vi "Analog Servo FPGA.vi"(9 "stop":bool) -> (1 "Clock":bool, 2 "Position Command":fxp<+/-,32,32>)   [LabVIEW 2012]
uses:
  <vilib>/Platform/TimedLoop/XDataNode/timing_clust.ctl
  <vilib>/Platform/TimedLoop/XDataNode/nitl_modes.ctl
  <vilib>/Platform/TimedLoop/XDataNode/wakeup.ctl
  <vilib>/rvi/Emulation/niFpgaSctlEmulationRegisterWithScheduler.vi
  <vilib>/rvi/eio/common/nirviEmuTemplateMethod_errors.vi
  <vilib>/rvi/Emulation/niFpgaSctlEmulationScheduler.vi
  <vilib>/rvi/Emulation/niFpgaSctlEmulationGetInTimedLoop.vi
  <vilib>/rvi/Emulation/niFpgaSctlEmulationGlobalWrite.vi
  <vilib>/Platform/TimedLoop/XDataNode/XDataNode.xnode
  <vilib>/eio/EIONode/EIONode.xnode
  <vilib>/Platform/TimedLoop/XDataNode/XDNodeRunTimeDep.lvlib
panel:
  in  "Shutdown Signal":fxp<+/-,20,5>=2.5
  out "Position Measured (Deg)":i32
  in  "Debug Command":fxp<+/-,16,10>
  in  "Debug?":bool
  out "Position Chart":cluster{"Position Setpoint (Deg)":i32, i32}(graph)
  in  "PID Gains":T1={"Kp"=50, "Kd"=0, "Ki"=0, "ILim"=1000, "Kv"=0, "Vff"=0, "Aff"=0, "Td"=0}
  out "Position (Counts)":i32
  in  "Reset Enc":bool
  in  "Cts/Rev":i64=30000
  out "Velocity (Counts/Interval)":i32
  in  "Position Setpoint (Deg)":i32
  out "Encoder B":i16(graph)
  out "Encoder A":i16(graph)
  # "Check specs for encoder \ncalibration value.  The default \nvalue is a placeholder only!"
  # "Switching into Debug mode\nwill allow you to send the\ndebug command out"
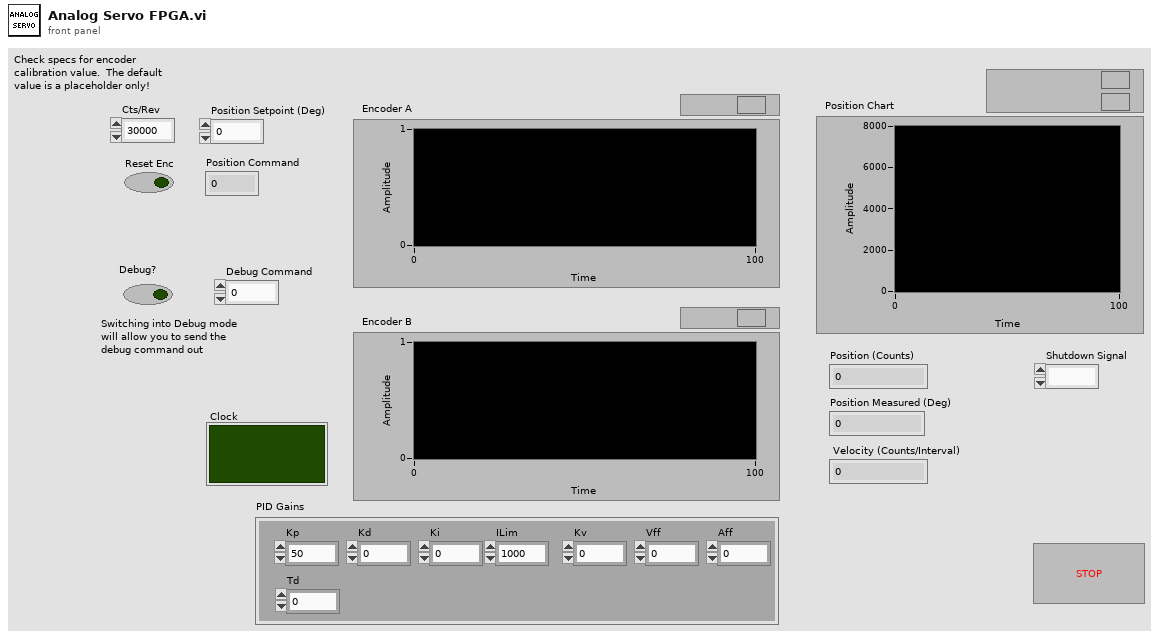
[diagram p1: front panel]
types:
  T1 = cluster{"Kp":i16, "Kd":i16, "Ki":i16, "ILim":i16, "Kv":i16, "Vff":i16, "Aff":i16, "Td":i16}
  T2 = typedef "XDNodeRunTimeDep.lvlib/timing_clust.ctl" = cluster{"Expected End [f-1]":u64, "Actual End [f-1]":u64, "Finished Late? [f-1]":bool, "Expected End [i-1]":u64, "Actual End [i-1]":u64, "Finished Late? [i-1]":bool, "Expected Start [i]":u64, "Actual Start [i]":u64, "Expected Start [f]":u64, "Actual Start [f]":u64, "Source Name":string, "Structure Name":string, "Period":i64, "Deadline":i64, "Offset":i64, "Start":i64, "Priority":i32, "Timeout":i32, "Mode":T3, "Wakeup Reason":T4, "Error":errorcluster, "Source Type":string, "Secondary Source Type":string, "Global End Time":u64, "Global Start Time":u64, "Frame Duration":u64, "Iteration Duration":u64, "Assigned CPU":i32, "I/O Scan Engine Mode":u32}
  T3 = typedef "XDNodeRunTimeDep.lvlib/nitl_modes.ctl" = enum32{"No Change", "Process missed periods, maintain original phase", "Discard missed periods, maintain original phase", "Process missed periods, ignore original phase", "Discard missed periods, ignore original phase"}
  T4 = typedef "XDNodeRunTimeDep.lvlib/wakeup.ctl" = enum32{"Normal", "Aborted", "Asynchronous wakeup", "Timing source error", "Timed loop error", "Timeout"}
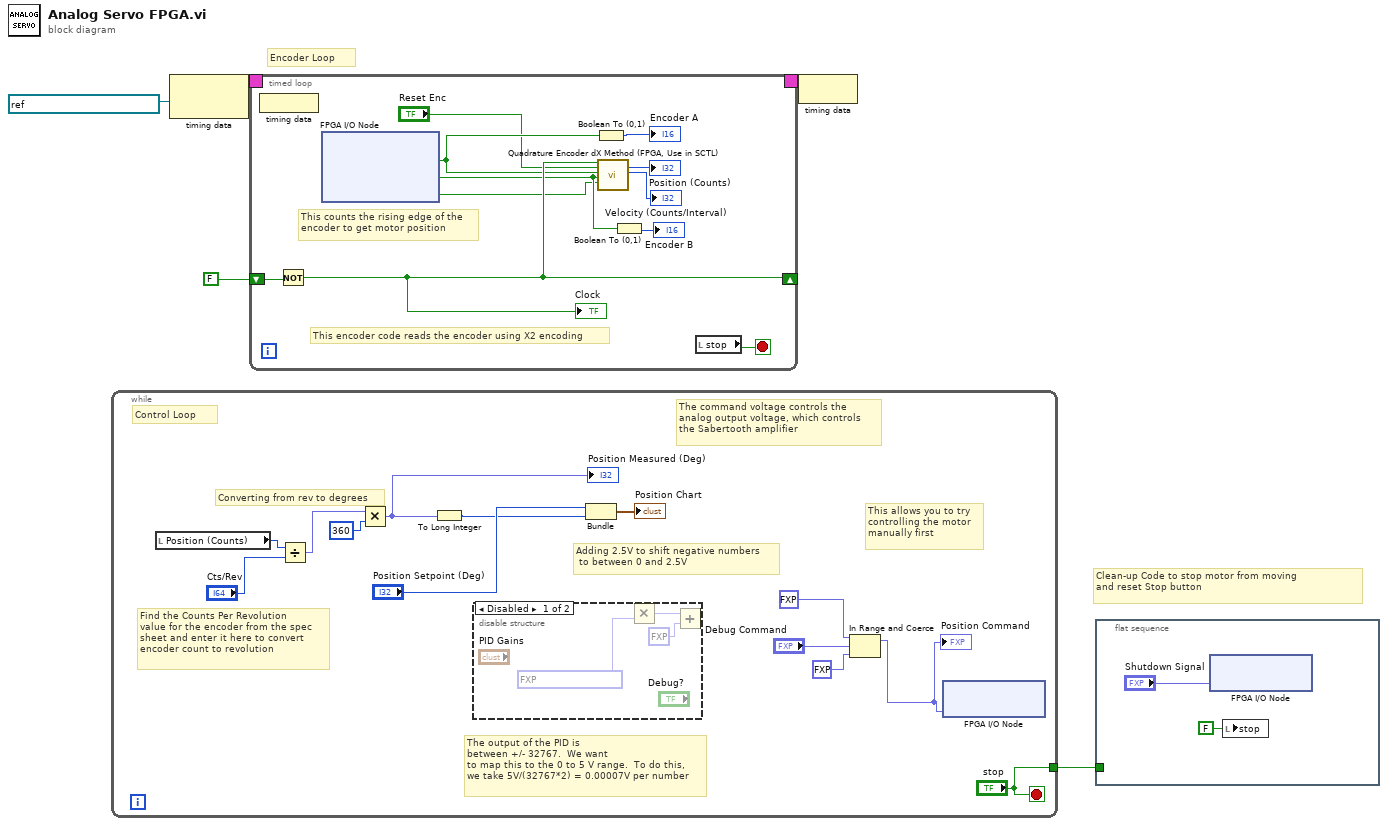
[diagram p0: block diagram]
diagram:
  # "Clean-up Code to stop motor from moving\nand reset Stop button"
  # "Encoder Loop"
  n1 = while {
    tunnel: ["stop"] -> w1
    stop <- "stop" stop-if-true
    # "Adding 2.5V to shift negative numbers\n to between 0 and 2.5V"
    # "Find the Counts Per Revolution\nvalue for the encoder from the spec\nsheet and enter it here to convert\nencoder count to revolution"
    # "The output of the PID is \nbetween +/- 32767.  We want\nto map this to the 0 to 5 V range.  To do this,\nwe take 5V/(32767*2) = 0.00007V per number"
    # "Control Loop"
    # "This allows you to try\ncontrolling the motor\nmanually first"
    # "Converting from rev to degrees"
    # "The command voltage controls the \nanalog output voltage, which controls\nthe Sabertooth amplifier"
    n2 = local read "Position (Counts)"() -> (w9:i32)
    n3 = Divide(x=w9, y="Cts/Rev") -> (x/y=w17:fxp<+/-,32,16>)
    n4 = Multiply(x=w17, y=360) -> (x*y=w8:fxp<+/-,64,48>)
    "Position Measured (Deg)" <- w8
    n5 = To Long Integer(number=w8) -> (32bit integer=w7:i32)
    n6 = disable-structure shown="Disabled" {
      frame Disabled {
        n7 = Multiply(y=fxp<+,18,1> 0.000762939453125) -> (x*y=w20:fxp<+,36,2>)  [unwired: 1 in]
        n8 = Add(x=w20, y=fxp<+/-,34,17> 2.5) -> ()  [unwired: 1 out]
      }
      frame Enabled {
      }
    }
    n9 = Bundle("Position Setpoint (Deg)"="Position Setpoint (Deg)", w7) -> (→"Position Chart":cluster{"Position Setpoint (Deg)":i32, i32})  [unwired: 1 in]
    n10 = In Range and Coerce(upper limit=fxp<+,3,3> 5.0, x="Debug Command", lower limit=fxp<+,1,1> 0.0) -> (coerced(x)=w6:fxp<+/-,16,10>)  [unwired: 1 out]
    "Position Command" <- w6
    n11 = xnode "FPGA I/O Node"("Servo Drive"=w6) -> ()  [unwired: 1 in, 1 out]
  }
  n12 = node-c288(refnum<k21> "40 MHz Onboard Clock" ("Source Name")) -> (w4:T2)
  n13 = timed-loop {
    timing: w4 -> [_]
    timing-out: [_] -> w3
    shift-right: [w31] -> _
    shift-left: FALSE -> [w32]
    stop <- w22 stop-if-true
    # "This encoder code reads the encoder using X2 encoding"
    # "This counts the rising edge of the\nencoder to get motor position"
    n14 = node-c288() -> ()  [unwired: 1 in]
    n15 = Not(x=w32) -> (.not. x?=w31:bool)
    "Clock" <- w31
    n16 = xnode "FPGA I/O Node"() -> ("Encoder A"=w30:bool, "Encoder B"=w29:bool, "Encoder Index"=w26:bool)  [unwired: 3 in, 3 out]
    n17 = Boolean To (0,1)(Boolean=w30) -> (0, 1=→"Encoder A":i16)
    n18 = call "Quadrature Encoder dX Method (FPGA, Use in SCTL).vi"("Clock"=w31, "Reset Enc"="Reset Enc", "A"=w30, "B"=w29, "Z"=w26) -> ("Position (Counts)"=→"Position (Counts)":i32, "Velocity (Counts/Interval)"=→"Velocity (Counts/Interval)":i32)  [unwired: 9 in, 4 out]
    n19 = Boolean To (0,1)(Boolean=w29) -> (0, 1=→"Encoder B":i16)
    n20 = local read "stop"() -> (w22:bool)
  }
  n21 = node-c288(w3) -> ()
  n22 = flat-sequence {
    tunnel: w1 -> [_]
    frame #0 {
      n23 = xnode "FPGA I/O Node"("Servo Drive"="Shutdown Signal") -> ()  [unwired: 1 in, 1 out]
      n24 = local write "stop"(FALSE ("stop")) -> ()
    }
  }
